vi "PH_PP_Common.get PSU Tagname.vi"(1 "PSU Tag":T2, 3 "PU":T1) -> (0 "PSU Tagname":string)   [LabVIEW 2014, in "PH_PP_Common.lvlib"]
doc: "This VI concatenates a Tagname out of strict type def enum controls. It keeps also the information whether the Tag is existing (if not, N/A is given out as name)."
uses:
  PH_PP_Common.lvlib
  PH_PP_Common.PSU Tags.ctl
  PH_PP_Common.PUs.ctl
  PH_PP_Common.Devices.ctl
  PH_Common/Names/PH_Names.Subsystems.ctl
  PH_Common/Names/PH_Names.Communication Type.ctl
  PH_Common/PH_Common.lvlib
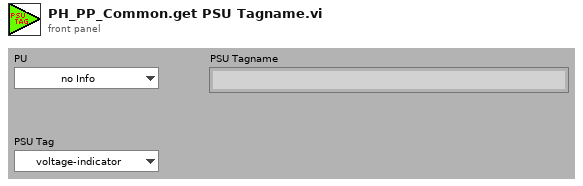
[diagram p1: front panel]
types:
  T1 = typedef "PH_PP_Common.lvlib/PH_PP_Common.PUs.ctl" = enum16{"no Info", "PA-19mm-1", "PA-19mm-2", "PA-45mm-PILC", "PA-45mm-MAIN", "MA-PU-1", "MA-PU-2", "MA-PU-3", "MA-PU-4", "MA-PU-5", "MA-PU-6", "MA-FR", "MA-PILC", "PA-45mm-DP"}
  T2 = typedef "PH_PP_Common.lvlib/PH_PP_Common.PSU Tags.ctl" = enum16{"voltage-indicator", "peak-detect", "current", "voltage", "inihibit-indicator", "end-of-charge", "HV-on-indicator", "overtemperature", "interlock-indicator", "load-fault", "sum-fault", "HV-off-indicator", "DC-ok", "inhibit", "HV-on", "interlock", "reset", "Status", "Limits"}
  T3 = typedef "PH_PP_Common.lvlib/PH_PP_Common.PSU Type.ctl" = enum16{"none", "Maxwell Standard", "DEL", "Maxwell ALE", "Continuum 601k"}
  T4 = typedef "PH_Common.lvlib/PH_Names.Subsystems.ctl" = enum16{"no Info", "fs-FE", "ns-FE", "PA", "MA", "MAS", "COS", "Exp-LB", "Exp-LL", "PP", "PILS"}
  T5 = typedef "PH_PP_Common.lvlib/PH_PP_Common.Devices.ctl" = enum16{"no Info", "Igni", "RR", "DumpRoss", "PSU", "Trigger", "HV-Meas", "Rods", "Chiller", "Conductivity", "Mercury"}
  T6 = typedef "PH_Common.lvlib/PH_Names.Communication Type.ctl" = enum16{"no Info", "SE", "SA", "AE", "AA", "DE", "DA", "DIM"}
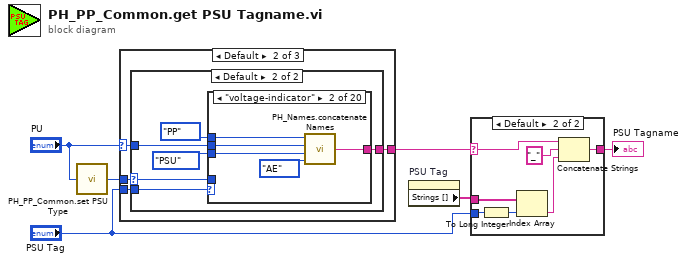
[diagram p0: block diagram]
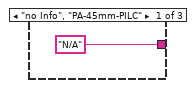
[diagram p2: hidden frame]
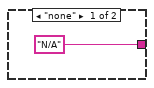
[diagram p3: hidden frame]
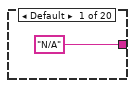
[diagram p4: hidden frame]
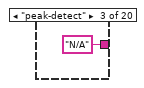
[diagram p5: hidden frame]
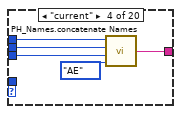
[diagram p6: hidden frame]
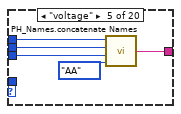
[diagram p7: hidden frame]
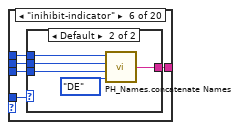
[diagram p8: hidden frame]
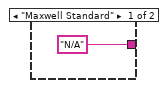
[diagram p9: hidden frame]
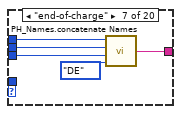
[diagram p10: hidden frame]
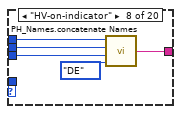
[diagram p11: hidden frame]
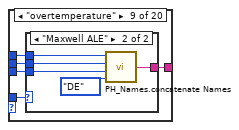
[diagram p12: hidden frame]
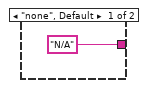
[diagram p13: hidden frame]
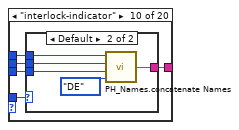
[diagram p14: hidden frame]
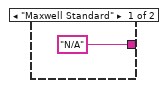
[diagram p15: hidden frame]
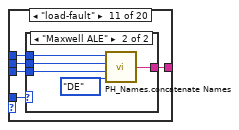
[diagram p16: hidden frame]
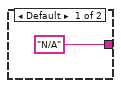
[diagram p17: hidden frame]
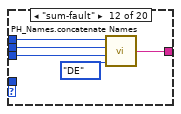
[diagram p18: hidden frame]
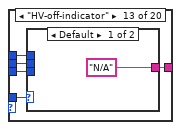
[diagram p19: hidden frame]
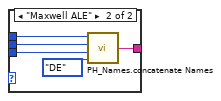
[diagram p20: hidden frame]
diagram:
  n1 = call "PH_PP_Common.set PSU Type.vi"("PU"="PU") -> ("PSU Type"=w1:T3)
  n2 = case shown="Default" "PU" {
    selector: "PU" -> [_ w8 w153]
    tunnel: ["N/A" ("Subsystem_PU_Devices_Comm Type") w11 w156] -> w5
    tunnel: w1 -> [_ w10 w155]
    tunnel: "PSU Tag" -> [_ w9 w154]
    frame "no Info", "PA-45mm-PILC" {
    }
    frame Default {
      n3 = case shown="Default" w10 {
        selector: w10 -> [_ w13]
        tunnel: ["N/A" ("Subsystem_PU_Devices_Comm Type") w18] -> w11
        tunnel: w8 -> [_ w17]
        tunnel: w9 -> [_ w15]
        frame "none" {
        }
        frame Default {
          n4 = case shown="\"voltage-indicator\"" w15 {
            tunnel: ["N/A" ("Subsystem_PU_Devices_Comm Type") w22 "N/A" ("Subsystem_PU_Devices_Comm Type") w28 w33 w39 w50 w55 w60 w71 w82 w93 w98 w109 w120 w125 w130 w135 w146 w151] -> w18
            tunnel: w17 -> [_ w21 _ w27 w32 w38 w49 w54 w59 w70 w81 w92 w97 w108 w119 w124 w129 w134 w145 w150]
            tunnel: PH_PP_Common.Devices."PSU" ("Devices (no info)") -> [_ w20 _ w26 w31 w37 w48 w53 w58 w69 w80 w91 w96 w107 w118 w123 w128 w133 w144 w149]
            tunnel: PH_Names.Subsystems."PP" ("Subsystem") -> [_ w23 _ w29 w34 w40 w51 w56 w61 w72 w83 w94 w99 w110 w121 w126 w131 w136 w147 w152]
            tunnel: w13 -> [_ _ _ _ _ w36 _ _ w57 w68 w79 _ w95 w106 _ _ _ w132 _ _]
            frame Default {
            }
            frame "voltage-indicator" {
              n5 = call "PH_Names.concatenate Names.vi"("Communication Type (no info)"=PH_Names.Communication_Type."AE", "Devices (no info)"=w20, "PU (no info)"=w21, "Subsystem"=w23) -> ("Subsystem_PU_Devices_Comm Type"=w22:string)
            }
            frame "peak-detect" {
            }
            frame "current" {
              n6 = call "PH_Names.concatenate Names.vi"("Communication Type (no info)"=PH_Names.Communication_Type."AE", "Devices (no info)"=w26, "PU (no info)"=w27, "Subsystem"=w29) -> ("Subsystem_PU_Devices_Comm Type"=w28:string)
            }
            frame "voltage" {
              n7 = call "PH_Names.concatenate Names.vi"("Communication Type (no info)"=PH_Names.Communication_Type."AA", "Devices (no info)"=w31, "PU (no info)"=w32, "Subsystem"=w34) -> ("Subsystem_PU_Devices_Comm Type"=w33:string)
            }
            frame "inihibit-indicator" {
              n8 = case shown="Default" w36 {
                tunnel: w40 -> [_ w45]
                tunnel: ["N/A" ("Subsystem_PU_Devices_Comm Type") w44] -> w39
                tunnel: w38 -> [_ w43]
                tunnel: w37 -> [_ w42]
                frame "Maxwell Standard" {
                }
                frame Default {
                  n9 = call "PH_Names.concatenate Names.vi"("Communication Type (no info)"=PH_Names.Communication_Type."DE", "Devices (no info)"=w42, "PU (no info)"=w43, "Subsystem"=w45) -> ("Subsystem_PU_Devices_Comm Type"=w44:string)
                }
              }
            }
            frame "end-of-charge" {
              n10 = call "PH_Names.concatenate Names.vi"("Communication Type (no info)"=PH_Names.Communication_Type."DE", "Devices (no info)"=w48, "PU (no info)"=w49, "Subsystem"=w51) -> ("Subsystem_PU_Devices_Comm Type"=w50:string)
            }
            frame "HV-on-indicator" {
              n11 = call "PH_Names.concatenate Names.vi"("Communication Type (no info)"=PH_Names.Communication_Type."DE", "Devices (no info)"=w53, "PU (no info)"=w54, "Subsystem"=w56) -> ("Subsystem_PU_Devices_Comm Type"=w55:string)
            }
            frame "overtemperature" {
              n12 = case shown="\"Maxwell ALE\"" w57 {
                tunnel: w61 -> [_ w67]
                tunnel: ["N/A" ("Subsystem_PU_Devices_Comm Type") w66] -> w60
                tunnel: w59 -> [_ w65]
                tunnel: w58 -> [_ w64]
                frame "none", Default {
                }
                frame "Maxwell ALE" {
                  n13 = call "PH_Names.concatenate Names.vi"("Communication Type (no info)"=PH_Names.Communication_Type."DE", "Devices (no info)"=w64, "PU (no info)"=w65, "Subsystem"=w67) -> ("Subsystem_PU_Devices_Comm Type"=w66:string)
                }
              }
            }
            frame "interlock-indicator" {
              n14 = case shown="Default" w68 {
                tunnel: w72 -> [_ w78]
                tunnel: ["N/A" ("Subsystem_PU_Devices_Comm Type") w77] -> w71
                tunnel: w70 -> [_ w76]
                tunnel: w69 -> [_ w75]
                frame "Maxwell Standard" {
                }
                frame Default {
                  n15 = call "PH_Names.concatenate Names.vi"("Communication Type (no info)"=PH_Names.Communication_Type."DE", "Devices (no info)"=w75, "PU (no info)"=w76, "Subsystem"=w78) -> ("Subsystem_PU_Devices_Comm Type"=w77:string)
                }
              }
            }
            frame "load-fault" {
              n16 = case shown="\"Maxwell ALE\"" w79 {
                tunnel: w83 -> [_ w89]
                tunnel: ["N/A" ("Subsystem_PU_Devices_Comm Type") w88] -> w82
                tunnel: w81 -> [_ w87]
                tunnel: w80 -> [_ w86]
                frame Default {
                }
                frame "Maxwell ALE" {
                  n17 = call "PH_Names.concatenate Names.vi"("Communication Type (no info)"=PH_Names.Communication_Type."DE", "Devices (no info)"=w86, "PU (no info)"=w87, "Subsystem"=w89) -> ("Subsystem_PU_Devices_Comm Type"=w88:string)
                }
              }
            }
            frame "sum-fault" {
              n18 = call "PH_Names.concatenate Names.vi"("Communication Type (no info)"=PH_Names.Communication_Type."DE", "Devices (no info)"=w91, "PU (no info)"=w92, "Subsystem"=w94) -> ("Subsystem_PU_Devices_Comm Type"=w93:string)
            }
            frame "HV-off-indicator" {
              n19 = case shown="Default" w95 {
                tunnel: w99 -> [_ w105]
                tunnel: ["N/A" ("Subsystem_PU_Devices_Comm Type") w104] -> w98
                tunnel: w97 -> [_ w103]
                tunnel: w96 -> [_ w102]
                frame Default {
                }
                frame "Maxwell ALE" {
                  n20 = call "PH_Names.concatenate Names.vi"("Communication Type (no info)"=PH_Names.Communication_Type."DE", "Devices (no info)"=w102, "PU (no info)"=w103, "Subsystem"=w105) -> ("Subsystem_PU_Devices_Comm Type"=w104:string)
                }
              }
            }
            frame "DC-ok" {
              n21 = case shown="\"Maxwell ALE\"" w106 {
                tunnel: w110 -> [_ w116]
                tunnel: ["N/A" ("Subsystem_PU_Devices_Comm Type") w115] -> w109
                tunnel: w108 -> [_ w114]
                tunnel: w107 -> [_ w113]
                frame Default {
                }
                frame "Maxwell ALE" {
                  n22 = call "PH_Names.concatenate Names.vi"("Communication Type (no info)"=PH_Names.Communication_Type."DE", "Devices (no info)"=w113, "PU (no info)"=w114, "Subsystem"=w116) -> ("Subsystem_PU_Devices_Comm Type"=w115:string)
                }
              }
            }
            frame "inhibit" {
              n23 = call "PH_Names.concatenate Names.vi"("Communication Type (no info)"=PH_Names.Communication_Type."DA", "Devices (no info)"=w118, "PU (no info)"=w119, "Subsystem"=w121) -> ("Subsystem_PU_Devices_Comm Type"=w120:string)
            }
            frame "HV-on" {
              n24 = call "PH_Names.concatenate Names.vi"("Communication Type (no info)"=PH_Names.Communication_Type."DA", "Devices (no info)"=w123, "PU (no info)"=w124, "Subsystem"=w126) -> ("Subsystem_PU_Devices_Comm Type"=w125:string)
            }
            frame "interlock" {
              n25 = call "PH_Names.concatenate Names.vi"("Communication Type (no info)"=PH_Names.Communication_Type."DA", "Devices (no info)"=w128, "PU (no info)"=w129, "Subsystem"=w131) -> ("Subsystem_PU_Devices_Comm Type"=w130:string)
            }
            frame "reset" {
              n26 = case shown="\"DEL\"" w132 {
                tunnel: w136 -> [_ w142]
                tunnel: ["N/A" ("Subsystem_PU_Devices_Comm Type") w141] -> w135
                tunnel: w134 -> [_ w140]
                tunnel: w133 -> [_ w139]
                frame Default {
                }
                frame "DEL" {
                  n27 = call "PH_Names.concatenate Names.vi"("Communication Type (no info)"=PH_Names.Communication_Type."DA", "Devices (no info)"=w139, "PU (no info)"=w140, "Subsystem"=w142) -> ("Subsystem_PU_Devices_Comm Type"=w141:string)
                }
              }
            }
            frame "Status" {
              n28 = call "PH_Names.concatenate Names.vi"("Communication Type (no info)"=PH_Names.Communication_Type."DIM", "Devices (no info)"=w144, "PU (no info)"=w145, "Subsystem"=w147) -> ("Subsystem_PU_Devices_Comm Type"=w146:string)
            }
            frame "Limits" {
              n29 = call "PH_Names.concatenate Names.vi"("Communication Type (no info)"=PH_Names.Communication_Type."DIM", "Devices (no info)"=w149, "PU (no info)"=w150, "Subsystem"=w152) -> ("Subsystem_PU_Devices_Comm Type"=w151:string)
            }
          }
        }
      }
    }
    frame "PA-45mm-DP" {
      n30 = case shown="Default" w155 {
        selector: w155 -> [_ w158]
        tunnel: ["N/A" ("Subsystem_PU_Devices_Comm Type") w163] -> w156
        tunnel: w153 -> [_ w162]
        tunnel: w154 -> [_ w160]
        frame "none" {
        }
        frame Default {
          n31 = case shown="\"voltage\"" w160 {
            tunnel: ["N/A" ("Subsystem_PU_Devices_Comm Type") w167 w173] -> w163
            tunnel: w162 -> [_ w166 w172]
            tunnel: PH_PP_Common.Devices."PSU" ("Devices (no info)") -> [_ w165 w171]
            tunnel: PH_Names.Subsystems."PP" ("Subsystem") -> [_ w168 w174]
            tunnel: w158 -> [_ _ _]
            frame Default {
            }
            frame "voltage" {
              n32 = call "PH_Names.concatenate Names.vi"("Communication Type (no info)"=PH_Names.Communication_Type."no Info", "Devices (no info)"=w165, "PU (no info)"=w166, "Subsystem"=w168) -> ("Subsystem_PU_Devices_Comm Type"=w167:string)
            }
            frame "Limits" {
              n33 = call "PH_Names.concatenate Names.vi"("Communication Type (no info)"=PH_Names.Communication_Type."no Info", "Devices (no info)"=w171, "PU (no info)"=w172, "Subsystem"=w174) -> ("Subsystem_PU_Devices_Comm Type"=w173:string)
            }
          }
        }
      }
    }
  }
  n34 = property on="PSU Tag" class="Enum (strict)"() -> ("Strings []"=w4:string[])  [unwired: 2 in, 2 out]
  n35 = case shown="Default" w5 {
    selector: w5 -> [_ w176]
    tunnel: ["N/A" w182] -> w6
    tunnel: w4 -> [_ w181]
    tunnel: "PSU Tag" -> [_ w177]
    frame "", "N/A" {
    }
    frame Default {
      n36 = To Long Integer(number=w177) -> (32bit integer=w180:i32)
      n37 = Index Array(array=w181, index=w180) -> (element=w179:string)
      n38 = Concatenate Strings(w176, "_" ("string"), w179) -> (w182:string)
    }
  }
  "PSU Tagname" <- w6
